vi "engineeringUpdateList.vi"(8 "error in (no error)":errorcluster, 11 "Model in":refnum<class "Model.lvclass">) -> (0 "error out":errorcluster, 3 "Model out":refnum<class "Model.lvclass">)   [LabVIEW 2016, in "Model.lvclass"]
uses:
  Model.lvclass
  Model.lvclass/Model.ctl
  ILCCommunications/ILCCommunications.lvclass/ILCCommunications.ctl
  Common_RT_Modbus/ModbusBuffer/ModbusBuffer.lvclass/ModbusBuffer.ctl
  Common_RT_ILC/ILC/ILC.lvclass/ILC.ctl
  Common_RT_FAILC/FAILC/FAILC.lvclass/FAILC.ctl
  Common_RT_HPILC/HPILC/HPILC.lvclass/HPILC.ctl
  ILCCommunications/broadcastFAForce.vi
  ILCCommunications/broadcastHPSteps.vi
  Common_RT_Modbus/ModbusBuffer/setIndex.vi
  Common_RT_FAILC/FAILC/startBroadcastSetForceFrame.vi
  Common_RT_ILC/ILC/getILCData.vi
  Common_RT_FAILC/FAILC/populateBroadcastSetForceFrame.vi
  Common_RT_FAILC/FAILC/completeBroadcastSetForceFrame.vi
  Common_RT_HPILC/HPILC/startBroadcastStepMotorFrame.vi
  Common_RT_HPILC/HPILC/populateBroadcastStepMotorFrame.vi
  Common_RT_HPILC/HPILC/completeBroadcastStepMotorFrame.vi
  Common_RT_Modbus/ModbusBuffer/writeHeader.vi
  Common_RT_Modbus/ModbusBuffer/writeU8.vi
  Common_RT_FAILC/FAILC/determineSlewFlagValue.vi
  Common_RT_Modbus/ModbusBuffer/getIndex.vi
  Common_RT_Modbus/ModbusBuffer/writeI24.vi
  Common_RT_Modbus/ModbusBuffer/writeCRC.vi
  Common_RT_Modbus/ModbusBuffer/writeDelay.vi
  Common_RT_Modbus/ModbusBuffer/writeEndOfFrame.vi
  Common_RT_Modbus/ModbusBuffer/writeI8.vi
  Common_RT_Modbus/ModbusBuffer/writeByteInstruction.vi
  Common_RT_Modbus/ModbusBuffer/calculateCRC.vi
  Common_RT_FAILC/FAILC/FAILC.lvclass
  D:/Code/ts_M1M3Support/Common_RT_ILC/ILC/ILC.lvclass
  Common_RT_HPILC/HPILC/HPILC.lvclass
  Resources/FPGA/FPGA.lvclass
  ILCCommunications/ILCCommunications.lvclass
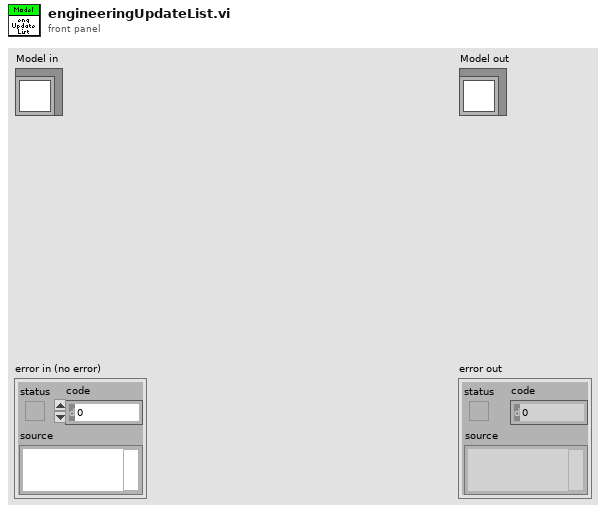
[diagram p1: front panel]
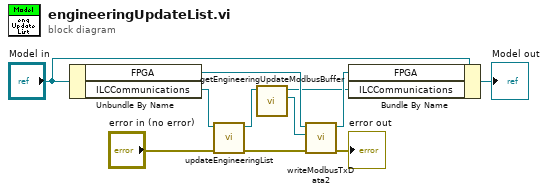
[diagram p0: block diagram]
diagram:
  n1 = Unbundle By Name("Model in") -> ("FPGA"=w11:refnum<class "FPGA.lvclass">, "ILCCommunications"=w6:refnum<class "ILCCommunications.lvclass">)
  n2 = call "updateEngineeringList.vi"("error in (no error)"="error in (no error)", "ILCCommunications in"=w6) -> ("error out"=w4:errorcluster, "ILCCommunications out"=w3:refnum<class "ILCCommunications.lvclass">)  [unwired: 8 in]
  n3 = call "getEngineeringUpdateModbusBuffer.vi"("ILCCommunications in"=w3) -> ("ModbusBuffer"=w1:refnum<class "ModbusBuffer.lvclass">, "ILCCommunications out"=w2:refnum<class "ILCCommunications.lvclass">)  [unwired: 9 in]
  n4 = call "writeModbusTxData2.vi"("error in (no error)"=w4, "ModbusBuffer in"=w1, "FPGA in"=w11) -> ("error out"=→"error out":errorcluster, "FPGA out"=w9:refnum<class "FPGA.lvclass">)  [unwired: 6 in, 1 out]
  n5 = Bundle By Name(cluster="Model in", "FPGA"=w9, "ILCCommunications"=w2) -> (→"Model out":refnum<class "Model.lvclass">)
